vi "SetupVoltageBase.vi"(0 "Refnum in":refnum<k21>, 1 "min":dbl, 2 "max":dbl, 3 "excitation value":dbl, 5 "physical channel":string, 9 "String":string, 11 "error in (no error)":errorcluster, 12 "voltage excitation source":i32(ring)=10200 items=["Internal"=10200, "External"=10167, "None"=10230], 13 "custom scale name":tag) -> (4 "Refnum out":refnum<k21>, 15 "error out":errorcluster)   [LabVIEW 2011]
uses:
  <vilib>/DAQmx/create/channels.llb/DAQmx Create Channel (AI-Voltage-Custom with Excitation).vi
  <vilib>/DAQmx/create/channels.llb/DAQmx Create Channel (TEDS-AI-Voltage-Custom with Excitation).vi
panel:
  in  "bridge configuration":i32(ring)=10228 items=["Full Bridge"=10182, "Half Bridge"=10187, "Quarter Bridge"=10270, "No Bridge"=10228]
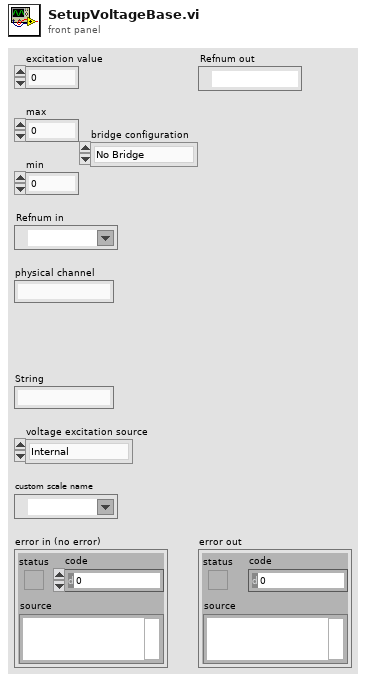
[diagram p1: front panel]
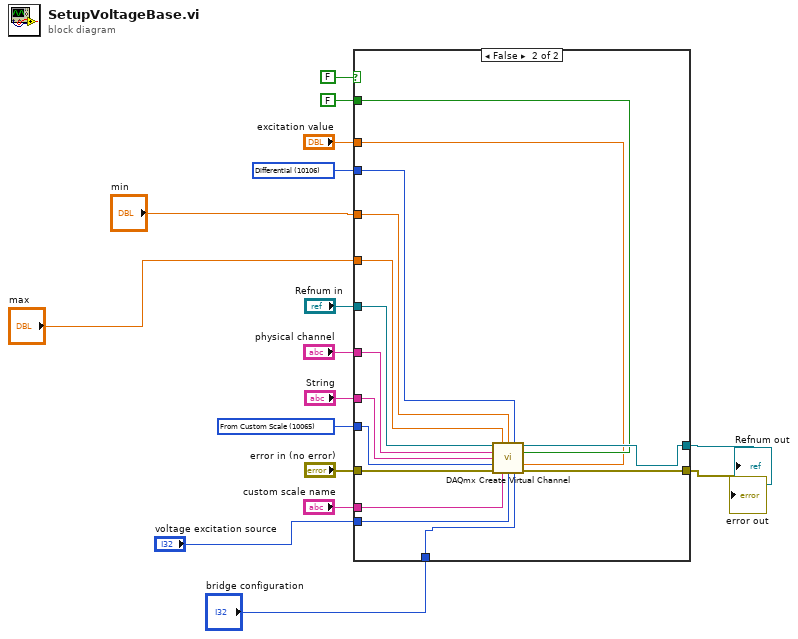
[diagram p0: block diagram]
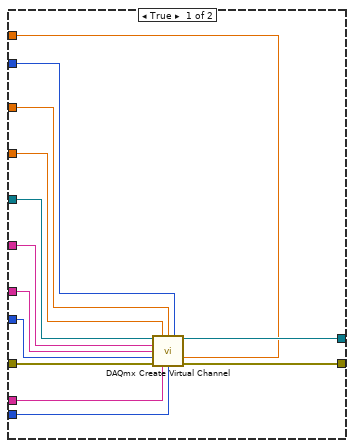
[diagram p2: hidden frame]
diagram:
  w3 = 10106 items=["default"=-1, "RSE"=10083, "NRSE"=10078, "Differential"=10106, "Pseudodifferential"=12529] ("input terminal configuration")
  w2 = 10065 items=["Volts"=10348, "From Custom Scale"=10065] ("units")
  n1 = case shown="False" FALSE {
    tunnel: "max" -> [w29 w44]
    tunnel: "min" -> [w28 w32]
    tunnel: w3 -> [w27 w43]
    tunnel: "Refnum in" -> [w26 w42]
    tunnel: "error in (no error)" -> [w25 w41]
    tunnel: [w24 w40] -> w15
    tunnel: [w23 w39] -> w16
    tunnel: "String" -> [w22 w38]
    tunnel: "physical channel" -> [w21 w37]
    tunnel: w2 -> [w20 w36]
    tunnel: "custom scale name" -> [w19 w35]
    tunnel: FALSE ("use excitation for scaling") -> [_ w34]
    tunnel: "excitation value" -> [w18 w33]
    tunnel: "voltage excitation source" -> [w17 w31]
    tunnel: "bridge configuration" -> [_ w30]
    frame True {
      n2 = call-poly <vilib>:"DAQmx Create Virtual Channel.vi"("task in"=w26, "maximum value"=w29, "minimum value"=w28, "input terminal configuration"=w27, "physical channels"=w21, "name to assign"=w22, "units"=w20, "voltage excitation value"=w18, "error in"=w25, "custom scale name"=w19, "voltage excitation source"=w17) -> ("task out"=w24:refnum<k21>, "error out"=w23:errorcluster)  [unwired: 2 in, 1 out]
    }
    frame False {
      n3 = call-poly <vilib>:"DAQmx Create Virtual Channel.vi"("task in"=w42, "maximum value"=w44, "minimum value"=w32, "input terminal configuration"=w43, "physical channels"=w37, "use excitation for scaling"=w34, "name to assign"=w38, "units"=w36, "voltage excitation value"=w33, "error in"=w41, "custom scale name"=w35, "voltage excitation source"=w31, "bridge configuration"=w30) -> ("task out"=w40:refnum<k21>, "error out"=w39:errorcluster)  [unwired: 1 out]
    }
  }
  "error out" <- w16
  "Refnum out" <- w15
